vi "Rohit_update time.vi"() -> ()   [LabVIEW 2009]
panel:
  out "date string":string
  out "time string":string
  out "current time":timestamp
  in  "?":bool
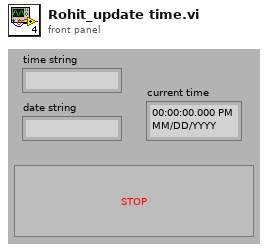
[diagram p1: front panel]
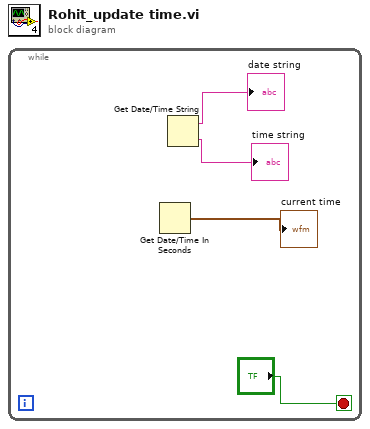
[diagram p0: block diagram]
diagram:
  n1 = while {
    stop <- "?" stop-if-true
    n2 = Get Date/Time In Seconds() -> (seconds since 1Jan1904=→"current time":timestamp)
    n3 = Get Date/Time String() -> (date string=→"date string":string, time string=→"time string":string)  [unwired: 3 in]
  }
